vi "Initialize Instrument.vi"(8 "error in (no error)":errorcluster, 10 "Reset":bool, 11 "VNA-ENA in":refnum<class "VNA-ENA.lvclass">) -> (0 "error out":errorcluster, 3 "VNA-ENA out":refnum<class "VNA-ENA.lvclass">)   [LabVIEW 2020, in "VNA-ENA.lvclass"]
uses:
  VNA-ENA.lvclass
  C:/Sandbox/Git_Sandbox/WiSpry Test Framework source code (LV20)/WiSpry Test Framework/Instruments/Instrument.lvclass
  C:/Sandbox/Git_Sandbox/WiSpry Test Framework source code (LV20)/WiSpry Test Framework/Instruments/Vector Network Analyzer/Vector Network Analyzer.lvclass
  <vilib>/Instr/_visa.llb/VISA Open Access Mode.ctl
  Instrument.lvclass/Instrument.ctl
  Vector Network Analyzer.lvclass/Vector Network Analyzer.ctl
  Instrument.lvclass
  Vector Network Analyzer.lvclass
  <instrlib>/Agilent ENA Series/Agilent ENA Series.lvlib
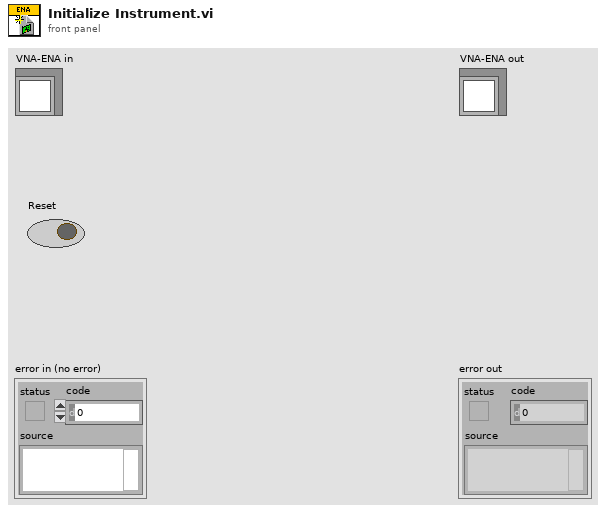
[diagram p1: front panel]
types:
  T1 = typedef "VISA Open Access Mode.ctl" = u32
  T2 = typedef "Instrument.lvclass/Interface String Cluster.ctl" = cluster{"Interface":string, "IDN string":string, "Instance":i32}
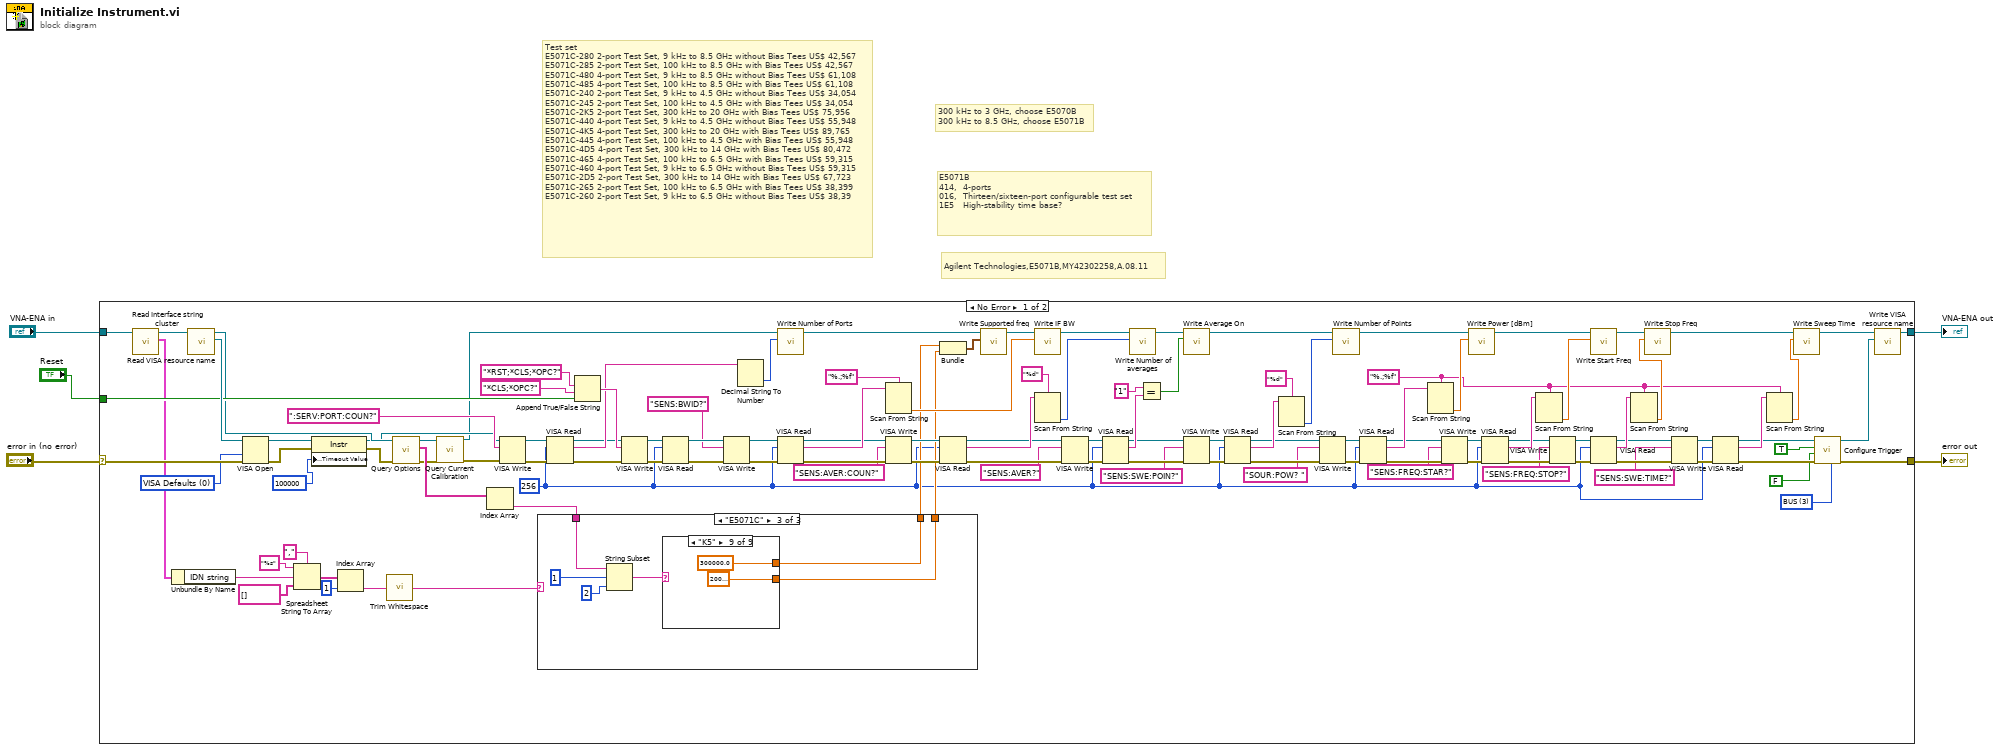
[diagram p0: block diagram]
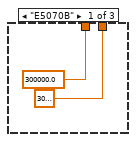
[diagram p2: hidden frame]
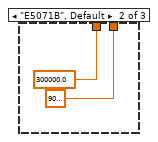
[diagram p3: hidden frame]
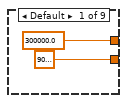
[diagram p4: hidden frame]
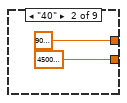
[diagram p5: hidden frame]
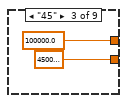
[diagram p6: hidden frame]
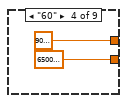
[diagram p7: hidden frame]
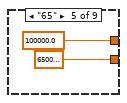
[diagram p8: hidden frame]
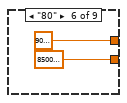
[diagram p9: hidden frame]
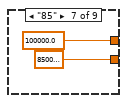
[diagram p10: hidden frame]
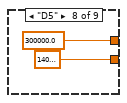
[diagram p11: hidden frame]
diagram:
  # "Agilent Technologies,E5071B,MY42302258,A.08.11"
  # "300 kHz to 3 GHz, choose E5070B\n300 kHz to 8.5 GHz, choose E5071B"
  # "E5071B\n414,  4-ports\n016,  Thirteen/sixteen-port configurable test set\n1E5   High-stability time base?"
  # "Test set\nE5071C-280\t2-port Test Set, 9 kHz to 8.5 GHz without Bias Tees\tUS$\t42,567\nE5071C-285\t2-port Test Set, 100 kHz to 8.5 GHz with Bias Tees\tUS$\t42,567\nE5071C-480\t4-port Test Set, 9 kHz to 8.5 GHz without Bias Tees\tUS$\t61,108\nE5071C-485\t4-port Test Set, 100 kHz to 8.5 GHz with Bias Tees\tUS$\t61,108\nE5071C-240\t2-port Test Set, 9 kHz to 4.5 GHz without Bias Tees\tUS$\t34,054\nE5071C-245\t2-port Test Set, 100 kHz to 4.5 GHz with Bias Tees\tUS$\t34,054\nE5071C-2K5\t2-port Test Set, 300 kHz to 20 GHz with Bias Tees\tUS$\t75,956\nE5071C-440\t4-port Test Set, 9 kHz to 4.5 GHz without Bias Tees\tUS$\t55,948\nE5071C-4K5\t4-port Test Set, 300 kHz to 20 GHz with Bias Tees\tUS$\t89,765\nE5071C-445\t4-port Test Set, 100 kHz to 4.5 GHz with Bias Tees\tUS$\t55,948\nE5071C-4D5\t4-port Test Set, 300 kHz to 14 GHz with Bias Tees\tUS$\t80,472\nE5071C-465\t4-port Test Set, 100 kHz to 6.5 GHz with Bias Tees\tUS$\t59,315\nE5071C-460\t4-port Test Set, 9 kHz to 6.5 GHz without Bias Tees\tUS$\t59,315\nE5071C-2D5\t2-port Test Set, 300 kHz to 14 GHz with Bias Tees\tUS$\t67,723\nE5071C-265\t2-port Test Set, 100 kHz to 6.5 GHz with Bias Tees\tUS$\t38,399\nE5071C-260\t2-port Test Set, 9 kHz to 6.5 GHz without Bias Tees\tUS$\t38,39"
  n1 = case shown="No Error" "error in (no error)" {
    selector: "error in (no error)" -> [w127 w156]
    tunnel: "VNA-ENA in" -> [w38 w157]
    tunnel: [w22 w156] -> w3
    tunnel: [w99 w157] -> w2
    tunnel: "Reset" -> [w42 _]
    frame No Error {
      w19 = u16 3 items=["Internal", "External", "Manual", "BUS"] ("Trigger Source (0: Internal)")
      w45 = "%.;%f" ("format string")
      w15 = u32 256 ("byte count")
      w125 = T1 0 items=["VISA Defaults"=0, "Exclusive Lock"=1, "Load Configured Settings"=4] ("Access Mode")
      n2 = call "Read Interface string cluster.vi"("Instrument in"=w38) -> ("Interface sting cluster"=w41:T2, "Instrument out"=w37:refnum<class "VNA-ENA.lvclass">)  [unwired: 9 in]
      n3 = Unbundle By Name(w41) -> ("IDN string"=w34:string)
      n4 = call "Read VISA resource name.vi"("Instrument in"=w37) -> ("VISA resource name"=w126:refnum<visa-resource-name>, "Instrument out"=w36:refnum<class "VNA-ENA.lvclass">)  [unwired: 9 in]
      n5 = VISA Open(access mode=w125, error in (no error)=w127, VISA resource name=w126) -> (VISA resource name=w123:refnum<visa-resource-name>, error out=w122:errorcluster)  [unwired: 2 in]
      n6 = Spreadsheet String To Array(delimiter (Tab)=",", format string="%s", spreadsheet string=w34, array type (2D Dbl)=string[] []) -> (array=w35:string[])
      n7 = property class="Instr"(reference=w123, error in=w122, "General Settings:Timeout Value"=u32 100000) -> (reference out=w10:refnum<visa-resource-name>, error out=w43:errorcluster)
      n8 = Index Array(array=w35, index=1) -> (element=w27:string)
      n9 = call <vilib>:"Trim Whitespace.vi"("string"=w27) -> ("trimmed string"=w26:string)  [unwired: 1 in]
      n10 = call-dynamic "Query Options.vi"("error in (no error)"=w43, "Instrument in"=w36) -> ("error out"=w7:errorcluster, "Options"=w29:string[], "Instrument out"=w9:refnum<class "VNA-ENA.lvclass">)  [unwired: 7 in]
      n11 = call-dynamic "Query Current Calibration.vi"("error in (no error)"=w7, "VNA-ENA in"=w9) -> ("error out"=w6:errorcluster, "VNA-ENA out"=w8:refnum<class "VNA-ENA.lvclass">)  [unwired: 8 in]
      n12 = Index Array(array=w29) -> (element=w16:string)  [unwired: 1 in]
      n13 = VISA Write(VISA resource name=w10, write buffer=":SERV:PORT:COUN?" ("Default Setup String"), error in (no error)=w6) -> (VISA resource name out=w18:refnum<visa-resource-name>, error out=w17:errorcluster)  [unwired: 1 out]
      n14 = case shown="\"E5071C\"" w26 {
        tunnel: [3000000000.0 9000000000.0 w137] -> w31
        tunnel: [300000.0 300000.0 w136] -> w30
        tunnel: w16 -> [_ _ w135]
        frame "E5070B" {
        }
        frame "E5071B", Default {
        }
        frame "E5071C" {
          n15 = String Subset(string=w135, offset (0)=1 ("length (rest)"), length (rest)=2 ("length (rest)")) -> (substring=w133:string)
          n16 = case shown="\"K5\"" w133 {
            tunnel: [9000000000.0 4500000000.0 4500000000.0 6500000000.0 6500000000.0 8500000000.0 8500000000.0 14000000000.0 20000000000.0] -> w137
            tunnel: [300000.0 9000.0 100000.0 9000.0 100000.0 9000.0 100000.0 300000.0 300000.0] -> w136
            frame Default {
            }
            frame "40" {
            }
            frame "45" {
            }
            frame "60" {
            }
            frame "65" {
            }
            frame "80" {
            }
            frame "85" {
            }
            frame "D5" {
            }
            frame "K5" {
            }
          }
        }
      }
      n17 = VISA Read(VISA resource name=w18, byte count=w15, error in (no error)=w17) -> (VISA resource name out=w11:refnum<visa-resource-name>, read buffer=w13:string, error out=w12:errorcluster)  [unwired: 1 out]
      n18 = Append True/False String(1:w42, 2:"*CLS;*OPC?" ("false string"), 3:"*RST;*CLS;*OPC?" ("Default Setup String")) -> (0:w119:string)  [unwired: 1 in]
      n19 = VISA Write(VISA resource name=w11, write buffer=w119, error in (no error)=w12) -> (VISA resource name out=w117:refnum<visa-resource-name>, error out=w118:errorcluster)  [unwired: 1 out]
      n20 = VISA Read(VISA resource name=w117, byte count=w15, error in (no error)=w118) -> (VISA resource name out=w106:refnum<visa-resource-name>, error out=w107:errorcluster)  [unwired: 2 out]
      n21 = VISA Write(VISA resource name=w106, write buffer="SENS:BWID?", error in (no error)=w107) -> (VISA resource name out=w108:refnum<visa-resource-name>, error out=w104:errorcluster)  [unwired: 1 out]
      n22 = Decimal String To Number(string=w13) -> (number=w28:i32)  [unwired: 2 in, 1 out]
      n23 = call "Write Number of Ports.vi"("Number of Ports"=w28, "Vector Network Analyzer in"=w8) -> ("Vector Network Analyzer out"=w116:refnum<class "VNA-ENA.lvclass">)  [unwired: 9 in]
      n24 = VISA Read(VISA resource name=w108, byte count=w15, error in (no error)=w104) -> (VISA resource name out=w97:refnum<visa-resource-name>, read buffer=w102:string, error out=w96:errorcluster)  [unwired: 1 out]
      n25 = Scan From String(format string="%.;%f", input string=w102) -> (output 1=w101:dbl)  [unwired: 3 in, 3 out]
      n26 = VISA Write(VISA resource name=w97, write buffer="SENS:AVER:COUN?", error in (no error)=w96) -> (VISA resource name out=w94:refnum<visa-resource-name>, error out=w98:errorcluster)  [unwired: 1 out]
      n27 = Bundle(w30, w31) -> (w115:cluster{dbl, dbl})  [unwired: 1 in]
      n28 = VISA Read(VISA resource name=w94, byte count=w15, error in (no error)=w98) -> (VISA resource name out=w88:refnum<visa-resource-name>, read buffer=w93:string, error out=w87:errorcluster)  [unwired: 1 out]
      n29 = call "Write Supported freq.vi"("Supported freq"=w115, "Vector Network Analyzer in"=w116) -> ("Vector Network Analyzer out"=w100:refnum<class "VNA-ENA.lvclass">)  [unwired: 9 in]
      n30 = call "Write IF BW.vi"("IF BW"=w101, "Vector Network Analyzer in"=w100) -> ("Vector Network Analyzer out"=w114:refnum<class "VNA-ENA.lvclass">)  [unwired: 9 in]
      n31 = Scan From String(format string="%d", input string=w93) -> (output 1=w91:i32)  [unwired: 3 in, 3 out]
      n32 = VISA Write(VISA resource name=w88, write buffer="SENS:AVER?", error in (no error)=w87) -> (VISA resource name out=w90:refnum<visa-resource-name>, error out=w89:errorcluster)  [unwired: 1 out]
      n33 = VISA Read(VISA resource name=w90, byte count=w15, error in (no error)=w89) -> (VISA resource name out=w80:refnum<visa-resource-name>, read buffer=w85:string, error out=w79:errorcluster)  [unwired: 1 out]
      n34 = call "Write Number of averages.vi"("Number of averages"=w91, "Vector Network Analyzer in"=w114) -> ("Vector Network Analyzer out"=w113:refnum<class "VNA-ENA.lvclass">)  [unwired: 9 in]
      n35 = Equal?(x="1", y=w85) -> (x = y?=w83:bool)
      n36 = call "Write Average On.vi"("Average On"=w83, "Vector Network Analyzer in"=w113) -> ("Vector Network Analyzer out"=w112:refnum<class "VNA-ENA.lvclass">)  [unwired: 9 in]
      n37 = VISA Write(VISA resource name=w80, write buffer="SENS:SWE:POIN?", error in (no error)=w79) -> (VISA resource name out=w81:refnum<visa-resource-name>, error out=w82:errorcluster)  [unwired: 1 out]
      n38 = VISA Read(VISA resource name=w81, byte count=w15, error in (no error)=w82) -> (VISA resource name out=w72:refnum<visa-resource-name>, read buffer=w76:string, error out=w71:errorcluster)  [unwired: 1 out]
      n39 = Scan From String(format string="%d", input string=w76) -> (output 1=w75:i32)  [unwired: 3 in, 3 out]
      n40 = VISA Write(VISA resource name=w72, write buffer="SOUR:POW? ", error in (no error)=w71) -> (VISA resource name out=w74:refnum<visa-resource-name>, error out=w73:errorcluster)  [unwired: 1 out]
      n41 = call "Write Number of Points.vi"("Number of Points"=w75, "Vector Network Analyzer in"=w112) -> ("Vector Network Analyzer out"=w111:refnum<class "VNA-ENA.lvclass">)  [unwired: 9 in]
      n42 = VISA Read(VISA resource name=w74, byte count=w15, error in (no error)=w73) -> (VISA resource name out=w65:refnum<visa-resource-name>, read buffer=w69:string, error out=w64:errorcluster)  [unwired: 1 out]
      n43 = Scan From String(format string=w45, input string=w69) -> (output 1=w68:dbl)  [unwired: 3 in, 3 out]
      n44 = VISA Write(VISA resource name=w65, write buffer="SENS:FREQ:STAR?", error in (no error)=w64) -> (VISA resource name out=w66:refnum<visa-resource-name>, error out=w67:errorcluster)  [unwired: 1 out]
      n45 = call "Write Power [dBm].vi"("Power [dBm]"=w68, "Vector Network Analyzer in"=w111) -> ("Vector Network Analyzer out"=w110:refnum<class "VNA-ENA.lvclass">)  [unwired: 9 in]
      n46 = VISA Read(VISA resource name=w66, byte count=w15, error in (no error)=w67) -> (VISA resource name out=w59:refnum<visa-resource-name>, read buffer=w62:string, error out=w58:errorcluster)  [unwired: 1 out]
      n47 = Scan From String(format string=w45, input string=w62) -> (output 1=w61:dbl)  [unwired: 3 in, 3 out]
      n48 = VISA Write(VISA resource name=w59, write buffer="SENS:FREQ:STOP?", error in (no error)=w58) -> (VISA resource name out=w60:refnum<visa-resource-name>, error out=w56:errorcluster)  [unwired: 1 out]
      n49 = call "Write Start Freq.vi"("Start Freq"=w61, "Vector Network Analyzer in"=w110) -> ("Vector Network Analyzer out"=w109:refnum<class "VNA-ENA.lvclass">)  [unwired: 9 in]
      n50 = VISA Read(VISA resource name=w60, byte count=w15, error in (no error)=w56) -> (VISA resource name out=w51:refnum<visa-resource-name>, read buffer=w54:string, error out=w50:errorcluster)  [unwired: 1 out]
      n51 = Scan From String(format string=w45, input string=w54) -> (output 1=w55:dbl)  [unwired: 3 in, 3 out]
      n52 = call "Write Stop Freq.vi"("Stop Freq"=w55, "Vector Network Analyzer in"=w109) -> ("Vector Network Analyzer out"=w48:refnum<class "VNA-ENA.lvclass">)  [unwired: 9 in]
      n53 = VISA Write(VISA resource name=w51, write buffer="SENS:SWE:TIME?", error in (no error)=w50) -> (VISA resource name out=w52:refnum<visa-resource-name>, error out=w53:errorcluster)  [unwired: 1 out]
      n54 = VISA Read(VISA resource name=w52, byte count=w15, error in (no error)=w53) -> (VISA resource name out=w24:refnum<visa-resource-name>, read buffer=w46:string, error out=w25:errorcluster)  [unwired: 1 out]
      n55 = Scan From String(format string=w45, input string=w46) -> (output 1=w44:dbl)  [unwired: 3 in, 3 out]
      n56 = call "Write Sweep Time.vi"("Sweep Time"=w44, "Vector Network Analyzer in"=w48) -> ("Vector Network Analyzer out"=w47:refnum<class "VNA-ENA.lvclass">)  [unwired: 9 in]
      n57 = call <instrlib>:"Configure Trigger.vi"("Trigger Source (0: Internal)"=w19, "error in (no error)"=w25, "Point Trigger (F: Disable)"=FALSE, "Continuous Sweep (T: Enable)"=TRUE, "VISA resource name"=w24) -> ("error out"=w22:errorcluster, "VISA resource name out"=w23:refnum<visa-resource-name>)  [unwired: 5 in]
      n58 = call "Write VISA resource name.vi"("VISA resource name"=w23, "Instrument in"=w47) -> ("Instrument out"=w99:refnum<class "VNA-ENA.lvclass">)  [unwired: 9 in]
    }
    frame Error {
    }
  }
  "error out" <- w3
  "VNA-ENA out" <- w2
